vi "HEWH 5 Minute SU0 Index.vi"(8 "error in (no error)":errorcluster, 10 "Test Data-Start to End DBL":dbl[][](array[numeric]), 11 "Draw Index in":i32[](array[numeric])) -> (0 "error out":errorcluster, 2 "TSUo Software Timestamp":dbl format="%#.6g", 3 "TSUo Index":i32)   [LabVIEW 2023]
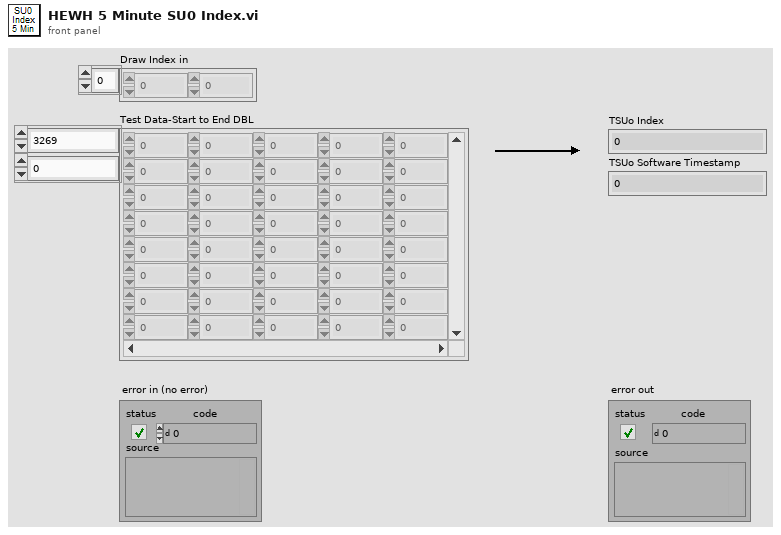
[diagram p1: front panel]
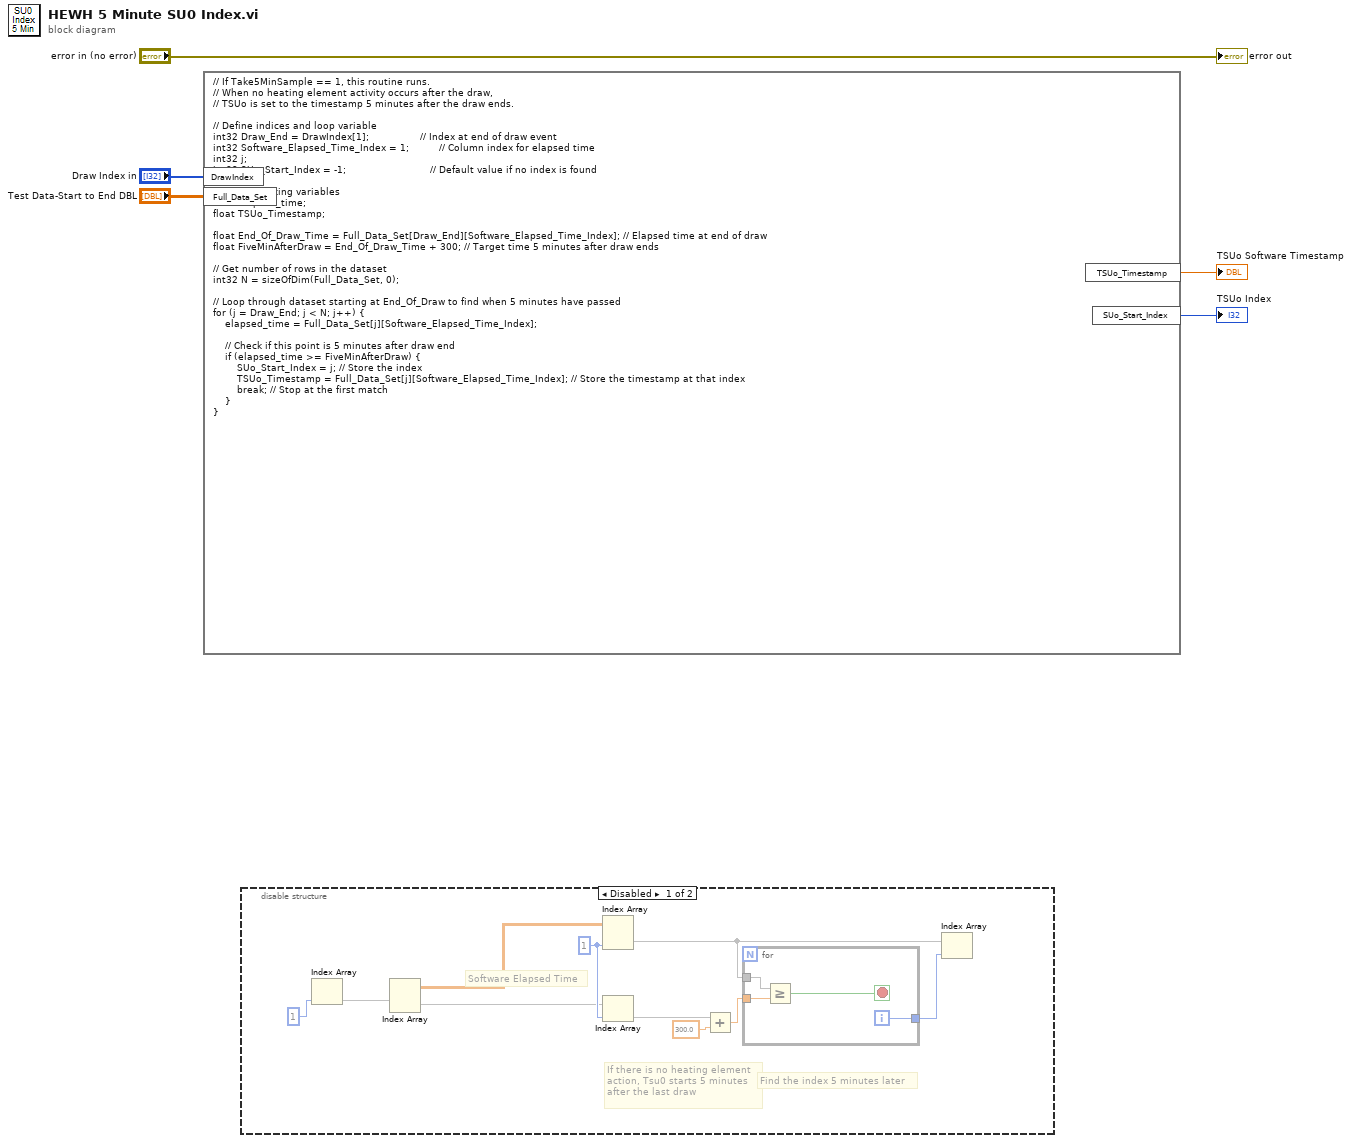
[diagram p0: block diagram]
diagram:
  n1 = formula code="// If Take5MinSample == 1, this routine runs.\n// When no heating element activity occurs after the draw,\n// TSUo is set to the timestamp 5 minutes after the draw ends.\n\n// Define indices and loop variable\nint32 Draw_End = DrawIndex[1];                 // Index at end of draw event\nint32 Software_Elapsed_Time_Index = 1;          // Column index for elapsed time\nint32 j;\nint32 SUo_Start_Index = -1;                            // Default value if no index is found\n\n// Define working variables\nfloat elapsed_time; \nfloat TSUo_Timestamp;\n\nfloat End_Of_Draw_Time = Full_Data_Set[Draw_End][Software_Elapsed_Time_Index]; // Elapsed time at end of draw\nfloat FiveMinAfterDraw = End_Of_Draw_Time + 300; // Target time 5 minutes after draw ends\n\n// Get number of rows in the dataset\nint32 N = sizeOfDim(Full_Data_Set, 0);\n\n// Loop through dataset starting at End_Of_Draw to find when 5 minutes have passed\nfor (j = Draw_End; j < N; j++) {\n    elapsed_time = Full_Data_Set[j][Software_Elapsed_Time_Index];\n\n    // Check if this point is 5 minutes after draw end\n    if (elapsed_time >= FiveMinAfterDraw) {\n        SUo_Start_Index = j; // Store the index\n        TSUo_Timestamp = Full_Data_Set[j][Software_Elapsed_Time_Index]; // Store the timestamp at that index\n        break; // Stop at the first match\n    }\n}"("Full_Data_Set"="Test Data-Start to End DBL", "DrawIndex"="Draw Index in") -> ("TSUo_Timestamp"=→"TSUo Software Timestamp":dbl, "SUo_Start_Index"=→"TSUo Index":i32)
  n2 = disable-structure shown="Disabled" {
    frame Disabled {
      w14 = 1 ("index")
      # "Find the index 5 minutes later"
      # "If there is no heating element\naction, Tsu0 starts 5 minutes\nafter the last draw"
      # "Software Elapsed Time"
      n3 = Index Array "Index Array"(index=1) -> (element=w13)  [unwired: 1 in]
      n4 = Index Array "Index Array"(index (row)=w13) -> (array=w6:dbl[][], element=w12)  [unwired: 1 in]
      n5 = Index Array "Index Array"(array=w6, index (col)=w14) -> (element=w15)  [unwired: 1 in]
      n6 = Index Array "Index Array"(array=w12, index=w14) -> (element=w9)
      n7 = Add(x=w9, y=300.0) -> (x+y=w11:dbl)
      n8 = for {
        tunnel: w11 -> [w16]
        tunnel: w15 -> [w17]
        tunnel: [w19] -> w7
        i -> [w19]
        stop <- w18 stop-if-true
        n9 = Greater Or Equal?(x=w17, y=w16) -> (x >= y?=w18:bool)
      }
      n10 = Index Array "Index Array"(array=w15, index=w7) -> ()  [unwired: 1 out]
    }
    frame Enabled {
    }
  }
  "error out" <- "error in (no error)"
